vi "6_1.vi"() -> ()   [LabVIEW 2017]
panel:
  out "路径":path
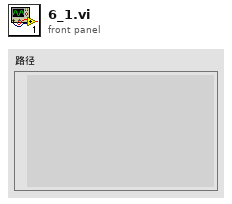
[diagram p1: front panel]
types:
  T1 = enum16{"open", "replace", "create", "open or create", "replace or create", "replace or create with confirmation"}
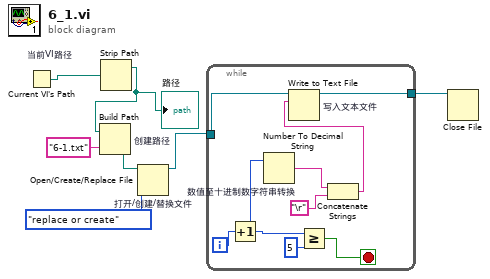
[diagram p0: block diagram]
diagram:
  n1 = Current VI's Path "当前VI路径"() -> (path=w2:path)
  n2 = Strip Path(path=w2) -> (stripped path=w1:path)  [unwired: 1 out]
  "路径" <- w1
  n3 = Build Path "创建路径"(base path=w1, name or relative path="6-1.txt" ("名称或相对路径")) -> (appended path=w5:path)
  n4 = Open/Create/Replace File "打开/创建/替换文件"(file path (use dialog)=w5, operation (0:open)=T1."replace or create" ("操作(0:open)")) -> (refnum out=w3:refnum<file>)  [unwired: 4 in, 2 out]
  n5 = while {
    tunnel: [w16] -> w4
    tunnel: w3 -> [w15]
    i -> [w11]
    stop <- w8 stop-if-true
    n6 = Increment(x=w11) -> (x+1=w9:i32)
    n7 = Number To Decimal String "数值至十进制数字符串转换"(number=w9) -> (decimal integer string=w14:string)  [unwired: 1 in]
    n8 = Greater Or Equal?(x=w9, y=5) -> (x >= y?=w8:bool)
    n9 = Concatenate Strings(w14, "\r") -> (w12:string)
    n10 = Write to Text File "写入文本文件"(file (use dialog)=w15, text=w12) -> (refnum out=w16:refnum<file>)  [unwired: 2 in, 2 out]
  }
  n11 = Close File(refnum=w4) -> ()  [unwired: 1 in, 2 out]
